vi "DCS_positioning.vi"(8 "error in (no error)":errorcluster, 9 "Data":dbl[](array[numeric])) -> (0 "X-Y position":dbl[](array[numeric]))   [LabVIEW 2012]
uses:
  <vilib>/Utility/file.llb/Read From Spreadsheet File (DBL).vi
panel:
  out "Simulated array dimensions":i32[](array[numeric])
  out "output array":dbl[][](array[numeric])
  out "all rows":dbl[][](array[numeric])
  in  "neg_neg_xy":path=path "C:/Users/Clavius/Documents/DCS/Simulation data/neg_neg_xy.csv"
  in  "neg_pos_xy":path=path "C:/Users/Clavius/Documents/DCS/Simulation data/neg_pos_xy.csv"
  in  "pos_pos_xy":path=path "C:/Users/Clavius/Documents/DCS/Simulation data/pos_pos_xy.csv"
  in  "pos_neg_xy":path=path "C:/Users/Clavius/Documents/DCS/Simulation data/pos_neg_xy.csv"
  out "min error":dbl
  in  "pos_neg":path=path "C:/Users/Clavius/Documents/DCS/Simulation data/pos_neg.csv"
  in  "pos_pos":path=path "C:/Users/Clavius/Documents/DCS/Simulation data/pos_pos.csv"
  in  "neg_neg":path=path "C:/Users/Clavius/Documents/DCS/Simulation data/neg_neg.csv"
  in  "neg_pos":path=path "C:/Users/Clavius/Documents/DCS/Simulation data/neg_pos.csv"
  # "Files"
  # "Information"
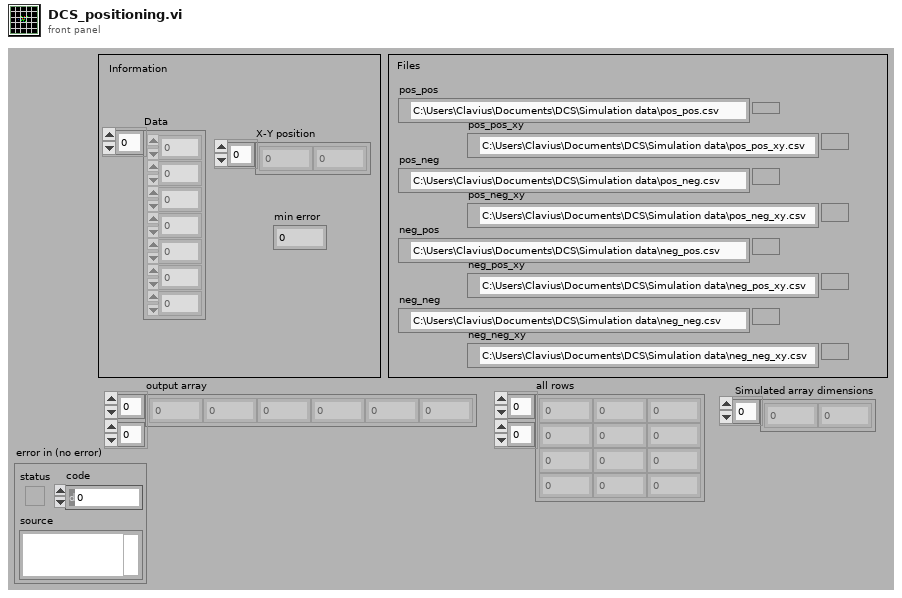
[diagram p1: front panel]
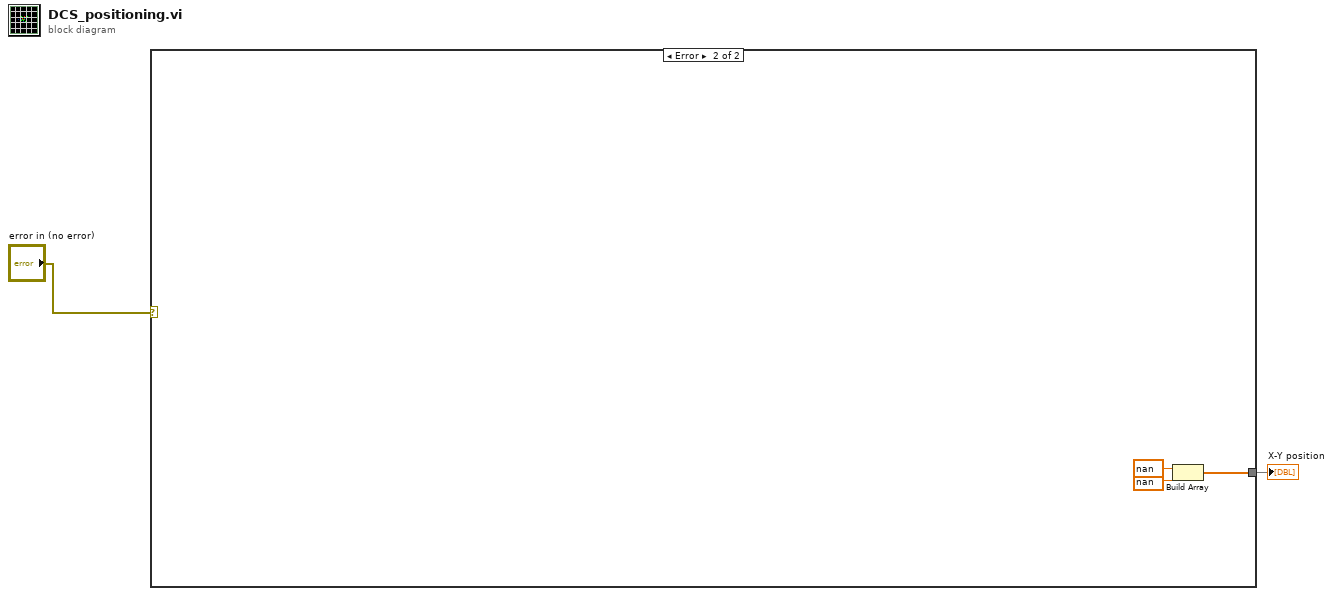
[diagram p0: block diagram]
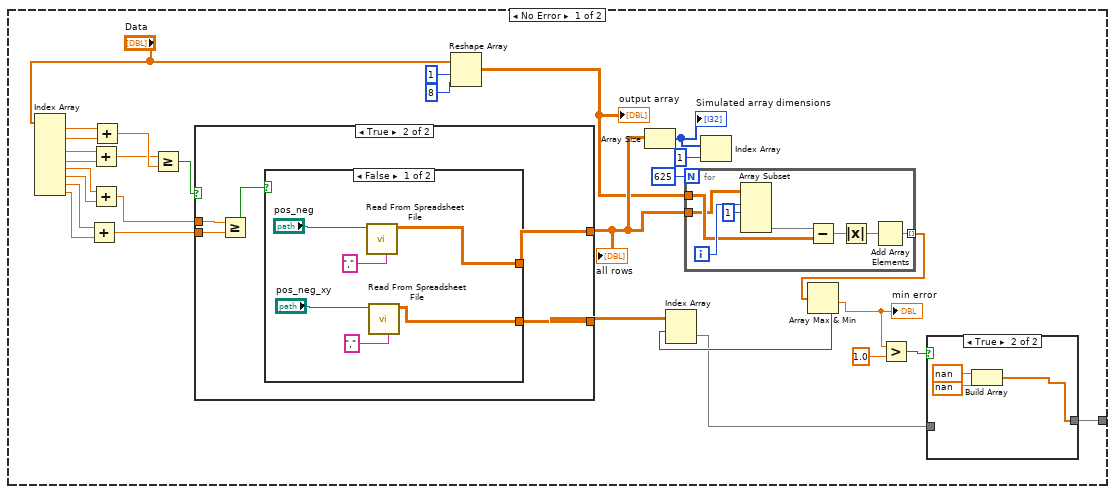
[diagram p2: hidden frame]
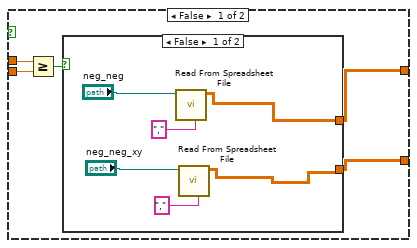
[diagram p4: hidden frame]
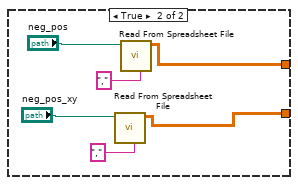
[diagram p5: hidden frame]
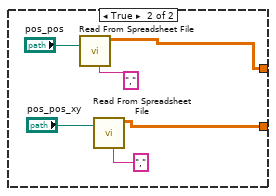
[diagram p6: hidden frame]
diagram:
  n1 = case shown="Error" "error in (no error)" {
    tunnel: [w4 w78] -> w2
    frame No Error {
      n2 = Index Array(array="Data") -> (element #1=w16:dbl, element #2=w17:dbl, element #3=w18:dbl, element #4=w19:dbl, element #5=w20:dbl, element #6=w21:dbl, element #7=w22:dbl, element #8=w23:dbl)  [unwired: 8 in]
      n3 = Add(x=w22, y=w23) -> (x+y=w27:dbl)
      n4 = Add(x=w18, y=w19) -> (x+y=w29:dbl)
      n5 = Add(x=w20, y=w21) -> (x+y=w28:dbl)
      n6 = Add(x=w16, y=w17) -> (x+y=w30:dbl)
      n7 = Greater Or Equal?(x=w29, y=w30) -> (x >= y?=w31:bool)
      n8 = case shown="True" w31 {
        tunnel: w28 -> [w48 w65]
        tunnel: w27 -> [w47 w64]
        tunnel: [w45 w62] -> w12
        tunnel: [w44 w61] -> w24
        frame False {
          n9 = Greater Or Equal?(x=w48, y=w47) -> (x >= y?=w46:bool)
          n10 = case shown="False" w46 {
            tunnel: [w50 w56] -> w45
            tunnel: [w49 w55] -> w44
            frame False {
              n11 = call-poly <vilib>:"Read From Spreadsheet File.vi"("delimiter (\\t)"="," ("delimiter (\\t)"), "file path (dialog if empty)"="neg_neg") -> ("all rows"=w50:dbl[][])  [unwired: 5 in, 4 out]
              n12 = call-poly <vilib>:"Read From Spreadsheet File.vi"("delimiter (\\t)"="," ("delimiter (\\t)"), "file path (dialog if empty)"="neg_neg_xy") -> ("all rows"=w49:dbl[][])  [unwired: 5 in, 4 out]
            }
            frame True {
              n13 = call-poly <vilib>:"Read From Spreadsheet File.vi"("delimiter (\\t)"="," ("delimiter (\\t)"), "file path (dialog if empty)"="neg_pos_xy") -> ("all rows"=w55:dbl[][])  [unwired: 5 in, 4 out]
              n14 = call-poly <vilib>:"Read From Spreadsheet File.vi"("delimiter (\\t)"="," ("delimiter (\\t)"), "file path (dialog if empty)"="neg_pos") -> ("all rows"=w56:dbl[][])  [unwired: 5 in, 4 out]
            }
          }
        }
        frame True {
          n15 = Greater Or Equal?(x=w65, y=w64) -> (x >= y?=w63:bool)
          n16 = case shown="False" w63 {
            tunnel: [w67 w73] -> w62
            tunnel: [w66 w72] -> w61
            frame False {
              n17 = call-poly <vilib>:"Read From Spreadsheet File.vi"("delimiter (\\t)"="," ("delimiter (\\t)"), "file path (dialog if empty)"="pos_neg") -> ("all rows"=w67:dbl[][])  [unwired: 5 in, 4 out]
              n18 = call-poly <vilib>:"Read From Spreadsheet File.vi"("delimiter (\\t)"="," ("delimiter (\\t)"), "file path (dialog if empty)"="pos_neg_xy") -> ("all rows"=w66:dbl[][])  [unwired: 5 in, 4 out]
            }
            frame True {
              n19 = call-poly <vilib>:"Read From Spreadsheet File.vi"("delimiter (\\t)"="," ("delimiter (\\t)"), "file path (dialog if empty)"="pos_pos") -> ("all rows"=w73:dbl[][])  [unwired: 5 in, 4 out]
              n20 = call-poly <vilib>:"Read From Spreadsheet File.vi"("delimiter (\\t)"="," ("delimiter (\\t)"), "file path (dialog if empty)"="pos_pos_xy") -> ("all rows"=w72:dbl[][])  [unwired: 5 in, 4 out]
            }
          }
        }
      }
      "all rows" <- w12
      n21 = Reshape Array("Data", 1 ("dimension size"), 8 ("dimension size")) -> (w9:dbl[][])
      "output array" <- w9
      n22 = Array Size(array=w12) -> (size(s)=w14:i32[])
      "Simulated array dimensions" <- w14
      n23 = for {
        N: 625 -> [_]
        tunnel: w9 -> [w37]
        tunnel: w12 -> [w36]
        tunnel: [w39] -> w11 mode=indexing
        i -> [w38]
        n24 = Array Subset(array=w36, index (row)=w38, length (row)=1 ("length")) -> (w40:dbl[][])  [unwired: 2 in]
        n25 = Subtract(x=w40, y=w37) -> (x-y=w42:dbl[][])
        n26 = Absolute Value(x=w42) -> (abs(x)=w41:dbl[][])
        n27 = Add Array Elements(numeric array=w41) -> (sum=w39:dbl)
      }
      n28 = Index Array(array=w14, index=1) -> ()  [unwired: 1 out]
      n29 = Array Max & Min(array=w11) -> (min value=w7:dbl, min index (indices)=w10:i32)  [unwired: 2 out]
      "min error" <- w7
      n30 = Index Array(array=w24, index (row)=w10) -> (element=w3:dbl[])  [unwired: 1 in]
      n31 = Greater?(x=w7, y=1.0) -> (0:w5:bool)
      n32 = case shown="True" w5 {
        tunnel: [w32 w33] -> w4
        tunnel: w3 -> [w32 _]
        frame False {
        }
        frame True {
          n33 = Build Array(nan ("element"), nan ("element")) -> (w33:dbl[])
        }
      }
    }
    frame Error {
      n34 = Build Array(nan ("element"), nan ("element")) -> (w78:dbl[])
    }
  }
  "X-Y position" <- w2
